vi "demonstrate cluster operations.vi"() -> ()   [LabVIEW 2013]
panel:
  out "Found 3":bool
  out "Found 2":bool
  out "ValueOut 2":i32
  out "ValueOut":i32
  out "Found":bool
  out "VElement":variant
  in  "Settings.StepSize":T1
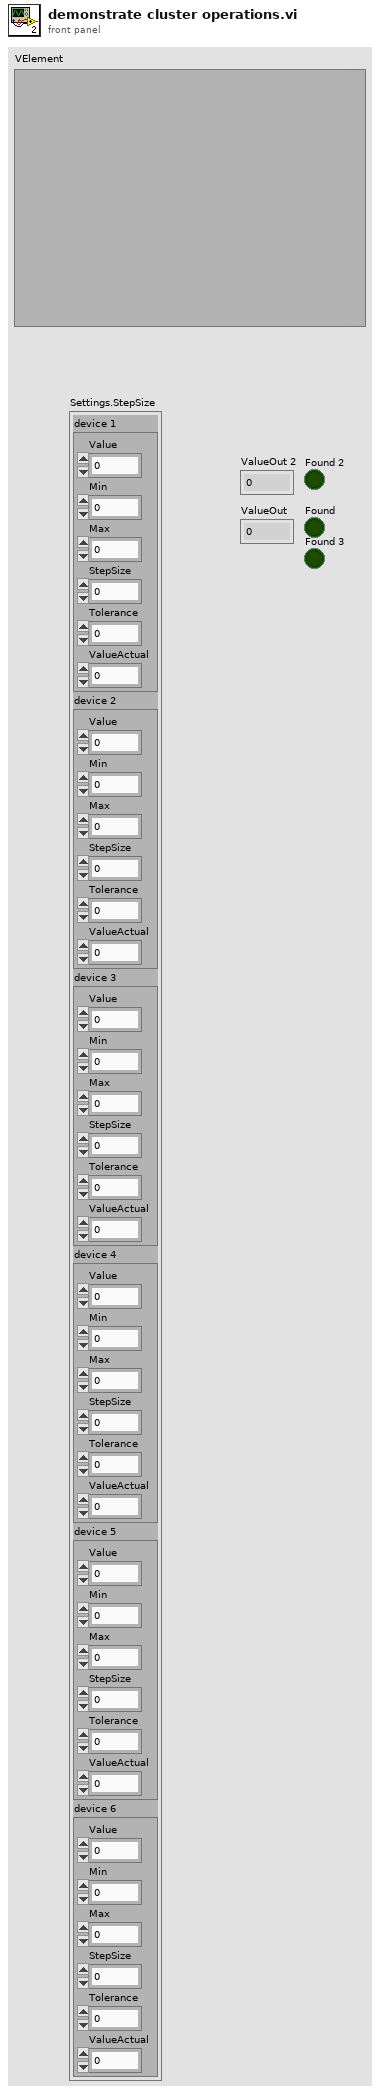
[diagram p1: front panel]
types:
  T1 = cluster{"device 1":cluster{"Value":dbl, "Min":dbl, "Max":dbl, "StepSize":dbl, "Tolerance":dbl, "ValueActual":dbl}, "device 2":cluster{"Value":dbl, "Min":dbl, "Max":dbl, "StepSize":dbl, "Tolerance":dbl, "ValueActual":dbl}, "device 3":cluster{"Value":dbl, "Min":dbl, "Max":dbl, "StepSize":dbl, "Tolerance":dbl, "ValueActual":dbl}, "device 4":cluster{"Value":dbl, "Min":dbl, "Max":dbl, "StepSize":dbl, "Tolerance":dbl, "ValueActual":dbl}, "device 5":cluster{"Value":dbl, "Min":dbl, "Max":dbl, "StepSize":dbl, "Tolerance":dbl, "ValueActual":dbl}, "device 6":cluster{"Value":dbl, "Min":dbl, "Max":dbl, "StepSize":dbl, "Tolerance":dbl, "ValueActual":dbl}}
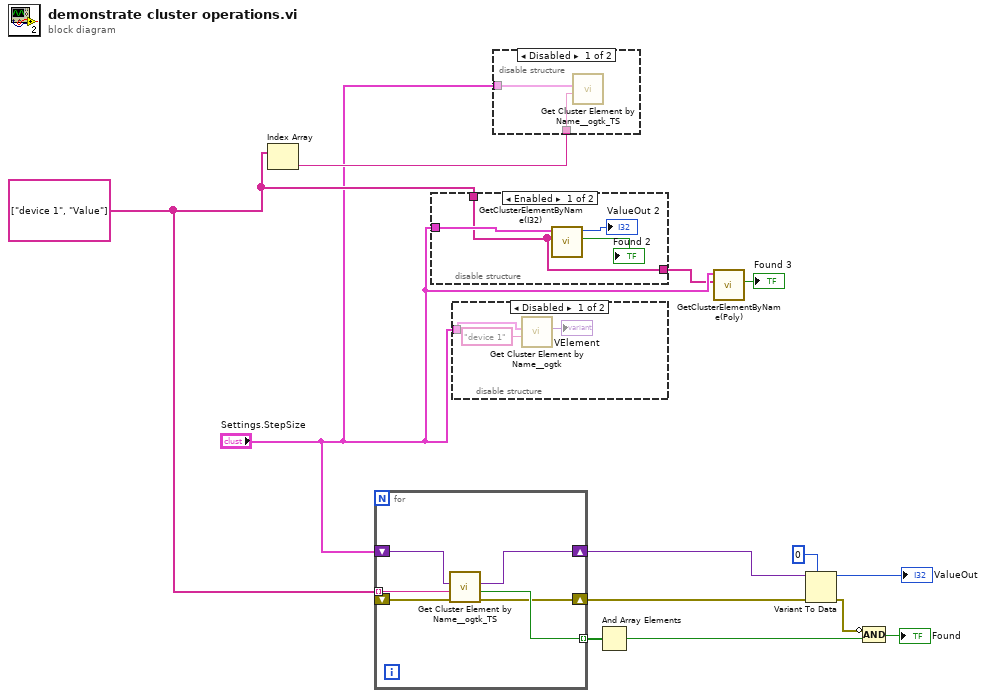
[diagram p0: block diagram]
diagram:
  w5 = string[] ["device 1", "Value"] ("ElementName")
  n1 = Index Array(array=w5) -> (element=w4:string)  [unwired: 1 in]
  n2 = for {
    tunnel: w5 -> [w19] mode=indexing
    shift-right: [w18] -> w12
    shift-left: "Settings.StepSize" -> [w17]
    tunnel: [w16] -> w13 mode=indexing
    shift-right: [w15] -> w10
    shift-left: _ -> [w14]
    n3 = call "Get Cluster Element by Name__ogtk_TS.vi"("error in (no error)"=w14, "Element Name"=w19, "Cluster"=w17) -> ("error out"=w15:errorcluster, "found?"=w16:bool, "VElement"=w18:variant)  [unwired: 6 in]
  }
  n4 = disable-structure shown="Enabled" {
    disable-tunnel: "Settings.StepSize" -> [w23 _]
    disable-tunnel: w5 -> [w20 _]
    disable-tunnel: [w20 _] -> w2
    frame Enabled {
      n5 = call "GetClusterElementByName(I32).vi"("ElementName"=w20, "VElement 2"=w23) -> ("Found"=→"Found 2":bool, "ValueOut"=→"ValueOut 2":i32)  [unwired: 8 in]
    }
    frame Disabled {
    }
  }
  n6 = disable-structure shown="Disabled" {
    disable-tunnel: "Settings.StepSize" -> [w25 _]
    frame Disabled {
      n7 = call <userlib>:"Get Cluster Element by Name__ogtk.vi"("Element Name"="device 1", "Cluster"=w25) -> ("VElement"=→"VElement":variant)  [unwired: 7 in, 2 out]
    }
    frame Enabled {
    }
  }
  n8 = disable-structure shown="Disabled" {
    disable-tunnel: "Settings.StepSize" -> [w28 _]
    disable-tunnel: w4 -> [w27 _]
    frame Disabled {
      n9 = call "Get Cluster Element by Name__ogtk_TS.vi"("Element Name"=w27, "Cluster"=w28) -> ()  [unwired: 7 in, 3 out]
    }
    frame Enabled {
    }
  }
  n10 = And Array Elements(Boolean array=w13) -> (logical AND=w9:bool)
  n11 = call-poly "GetClusterElementByName(Poly).vi"("ElementName"=w2, "VElement 2"="Settings.StepSize") -> ("Found"=→"Found 3":bool)  [unwired: 8 in, 1 out]
  n12 = Variant To Data(error in=w10, type=0, Variant=w12) -> (data=→"ValueOut":i32, error out=w7:errorcluster)
  n13 = Compound Arithmetic op=AND(invert w7, w9) -> (→"Found":bool)
